vi "wetter_main.vi"() -> ()   [LabVIEW 2018]
uses:
  <vilib>/National Instruments/Dark Sky Weather Data for LabVIEW/Dark Sky Weather Data for LabVIEW.lvlib
panel:
  out "Numeric":i32
  in  "stop":bool
  out "ozone":dbl
  out "pressure":dbl
  out "cloudCover":dbl
  out "visibility":dbl
  out "windBearing":dbl
  out "windGust":dbl
  out "windSpeed":dbl
  out "humidity":dbl
  out "dewPoint":dbl
  out "apparentTemp":dbl
  out "temperature":dbl
  out "precipType":string
  out "precipProbability":dbl
  out "PrecipIntensityError":dbl
  out "precipIntensity":dbl
  out "nearestStormDistance":dbl
  out "icon":string
  out "summary":string
  out "time":dbl
  in  "Get Weather":bool
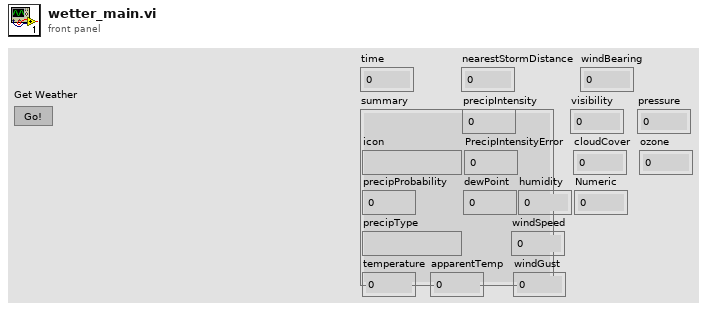
[diagram p1: front panel]
types:
  T1 = cluster{"Geographical Location":string, "Machine IP (As seen by geocoder)":string, "ISP":string, "Latitude":dbl, "Longitude":dbl, "Boolean":bool}
  T2 = typedef "Dark Sky Weather Data for LabVIEW.lvlib/Forecast Output.ctl" = cluster{"Lat, Long, Timezone":T3, "Current Data":T4, "Minutely Data":T5, "Hourly Data":T6, "Daily Data":T7, "Alerts":T8}
  T3 = typedef "Dark Sky Weather Data for LabVIEW.lvlib/Lat_Lon_TZ.ctl" = cluster{"latitude":dbl, "longitude":dbl, "timezone":string, "offset":dbl}
  T4 = typedef "Dark Sky Weather Data for LabVIEW.lvlib/Forecast Current Data.ctl" = cluster{"currently":cluster{"time":dbl, "summary":string, "icon":string, "nearestStormDistance":dbl, "precipIntensity":dbl, "PrecipIntensityError":dbl, "precipProbability":dbl, "precipType":string, "temperature":dbl, "apparentTemp":dbl, "dewPoint":dbl, "humidity":dbl, "windSpeed":dbl, "windGust":dbl, "windBearing":dbl, "visibility":dbl, "cloudCover":dbl, "pressure":dbl, "ozone":dbl}}
  T5 = typedef "Dark Sky Weather Data for LabVIEW.lvlib/Forecast Minutely Data.ctl" = cluster{"minutely":cluster{"summary":string, "icon":string, "data":cluster{"time":dbl, "precipIntensity":dbl, "precipIntensityError":dbl, "precipProbability":dbl, "precipType":string}[]}}
  T6 = typedef "Dark Sky Weather Data for LabVIEW.lvlib/Forecast Hourly Data.ctl" = cluster{"hourly":cluster{"summary":string, "icon":string, "data":cluster{"time":dbl, "summary":string, "icon":string, "precipIntensity":dbl, "precipProbability":dbl, "precipType":string, "temperature":dbl, "apparentTemp":dbl, "dewPoint":dbl, "humidity":dbl, "windSpeed":dbl, "windGust":dbl, "windBearing":dbl, "visibility":dbl, "cloudCover":dbl, "pressure":dbl, "ozone":dbl}[]}}
  T7 = typedef "Dark Sky Weather Data for LabVIEW.lvlib/Forecast Daily Data.ctl" = cluster{"daily":cluster{"summary":string, "icon":string, "data":cluster{"time":dbl, "summary":string, "icon":string, "sunriseTime":dbl, "sunsetTime":dbl, "moonPhase":dbl, "precipIntensity":dbl, "precipIntensityMax":dbl, "precipIntensityMaxTime":dbl, "precipProbability":dbl, "precipType":string, "temperatureMin":dbl, "temperatureMinTime":dbl, "temperatureMax":dbl, "temperatureMaxTime":dbl, "apparentTempMin":dbl, "apparentTempMinTime":dbl, "apparentTempMax":dbl, "apparentTempMaxTime2":dbl, "dewPoint":dbl, "humidity":dbl, "windSpeed":dbl, "windBearing":dbl, "visibility":dbl, "cloudCover":dbl, "pressure":dbl, "ozone":dbl}[]}}
  T8 = typedef "Dark Sky Weather Data for LabVIEW.lvlib/Forecast Alert Data.ctl" = cluster{"alerts":cluster{"title":string, "time":dbl, "expires":dbl, "description":string, "uri":string}[]}
  T9 = cluster{"time":dbl, "summary":string, "icon":string, "nearestStormDistance":dbl, "precipIntensity":dbl, "PrecipIntensityError":dbl, "precipProbability":dbl, "precipType":string, "temperature":dbl, "apparentTemp":dbl, "dewPoint":dbl, "humidity":dbl, "windSpeed":dbl, "windGust":dbl, "windBearing":dbl, "visibility":dbl, "cloudCover":dbl, "pressure":dbl, "ozone":dbl}
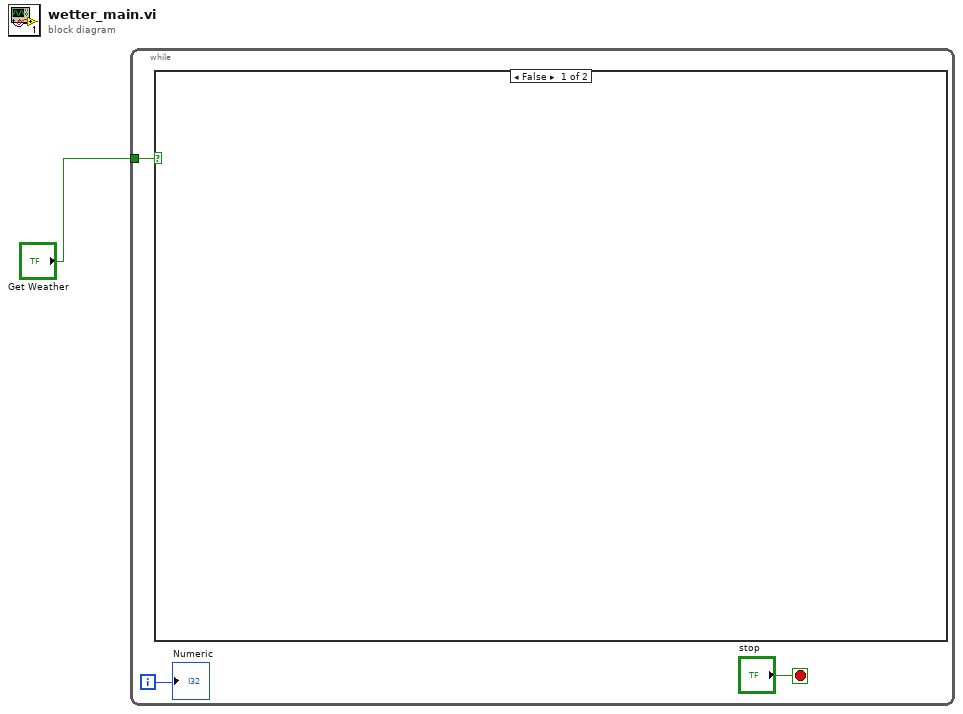
[diagram p0: block diagram]
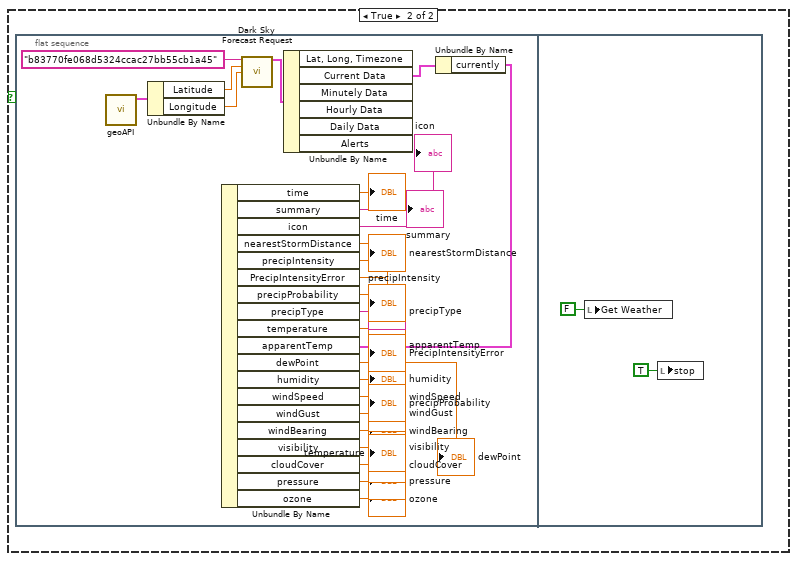
[diagram p2: hidden frame]
diagram:
  n1 = while {
    tunnel: "Get Weather" -> [w4]
    i -> [w2]
    stop <- "stop" stop-if-true
    n2 = case shown="False" w4 {
      frame False {
      }
      frame True {
        n3 = flat-sequence {
          frame #0 {
            n4 = call "geoAPI.vi"() -> ("Cluster 2"=w30:T1)  [unwired: 11 in]
            n5 = Unbundle By Name(w30) -> ("Latitude"=w29:dbl, "Longitude"=w28:dbl)
            n6 = call <vilib>:"Dark Sky Forecast Request.vi"("API Key"="b83770fe068d5324ccac27bb55cb1a45", "Latitude"=w29, "Longitude"=w28) -> ("Forecast Output"=w26:T2)  [unwired: 11 in, 1 out]
            n7 = Unbundle By Name(w26) -> ("Current Data"=w25:T4)  [unwired: 5 out]
            n8 = Unbundle By Name(w25) -> ("currently"=w24:T9)
            n9 = Unbundle By Name(w24) -> ("time"=→"time":dbl, "summary"=→"summary":string, "icon"=→"icon":string, "nearestStormDistance"=→"nearestStormDistance":dbl, "precipIntensity"=→"precipIntensity":dbl, "PrecipIntensityError"=→"PrecipIntensityError":dbl, "precipProbability"=→"precipProbability":dbl, "precipType"=→"precipType":string, "temperature"=→"temperature":dbl, "apparentTemp"=→"apparentTemp":dbl, "dewPoint"=→"dewPoint":dbl, "humidity"=→"humidity":dbl, "windSpeed"=→"windSpeed":dbl, "windGust"=→"windGust":dbl, "windBearing"=→"windBearing":dbl, "visibility"=→"visibility":dbl, "cloudCover"=→"cloudCover":dbl, "pressure"=→"pressure":dbl, "ozone"=→"ozone":dbl)
          }
          frame #1 {
            n10 = local write "Get Weather"(FALSE ("Get Weather")) -> ()
            n11 = local write "stop"(TRUE ("stop")) -> ()
          }
        }
      }
    }
    "Numeric" <- w2
  }
